vi "09.Evd.4_Ask.3.vi"() -> ()   [LabVIEW 2025]
panel:
  out "Comparison Tries":dbl
  in  "Stop":bool
  out "Equality Found":bool
  out "B":dbl
  out "A":dbl
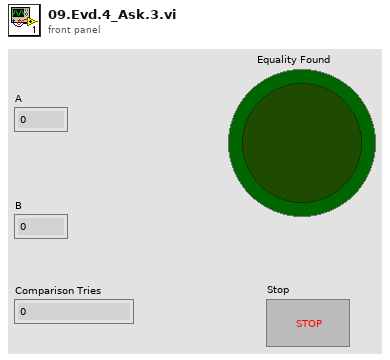
[diagram p1: front panel]
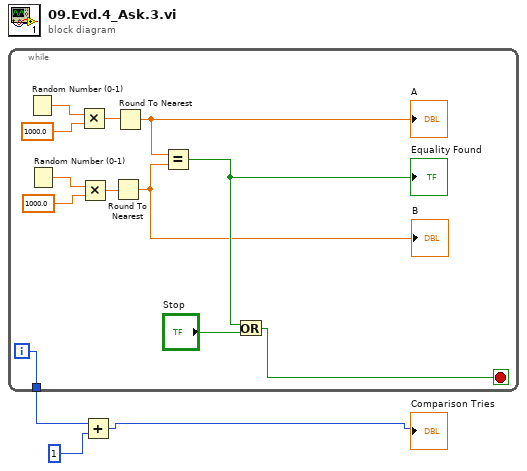
[diagram p0: block diagram]
diagram:
  n1 = while {
    tunnel: [w5] -> w2
    i -> [w5]
    stop <- w13 stop-if-true
    n2 = Random Number (0-1) ("Random Number (1-10)")() -> (number: 0 to 1=w12:dbl)
    n3 = Random Number (0-1) ("Random Number (1-10)")() -> (number: 0 to 1=w10:dbl)
    n4 = Multiply(x=w12, y=1000.0) -> (x*y=w8:dbl)
    n5 = Multiply(x=w10, y=1000.0) -> (x*y=w7:dbl)
    n6 = Round To Nearest(number=w7) -> (nearest integer value=w6:dbl)
    "B" <- w6
    n7 = Round To Nearest(number=w8) -> (nearest integer value=w4:dbl)
    "A" <- w4
    n8 = Equal?(x=w4, y=w6) -> (x = y?=w15:bool)
    "Equality Found" <- w15
    n9 = Or(x=w15, y="Stop") -> (x .or. y?=w13:bool)
  }
  n10 = Add(x=w2, y=1) -> (x+y=→"Comparison Tries":i32)
